vi "Create Image Saving Folder.vi"(0 "Camera Prime95B Controller in":refnum<class "Camera Prime95B Controller.lvclass">, 5 "Save Path":path, 7 "File suffix":string, 9 "StreamToDisk?":bool, 11 "error in (no error)":errorcluster) -> (4 "Camera Prime95B Controller out":refnum<class "Camera Prime95B Controller.lvclass">, 6 "Saving Path":path, 8 "Stream Saving Path":path, 15 "error out":errorcluster)   [LabVIEW 2020, in "Camera_Prime95B.lvlib" / "Camera Prime95B Controller.lvlib" / "Camera Prime95B Controller.lvclass"]
uses:
  Camera Prime95B Controller.lvclass
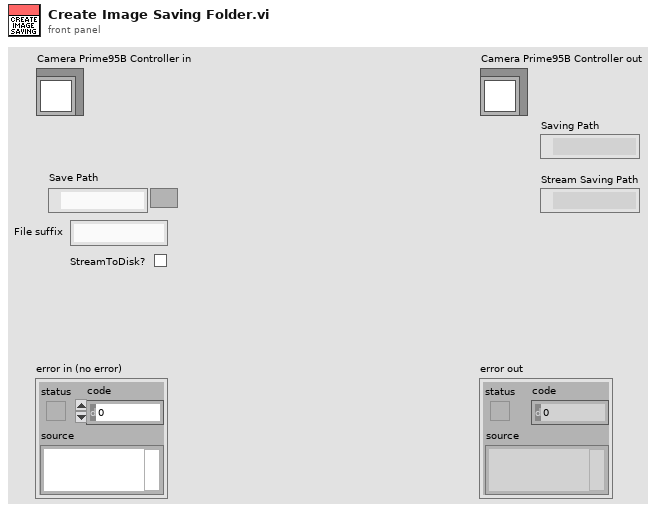
[diagram p1: front panel]
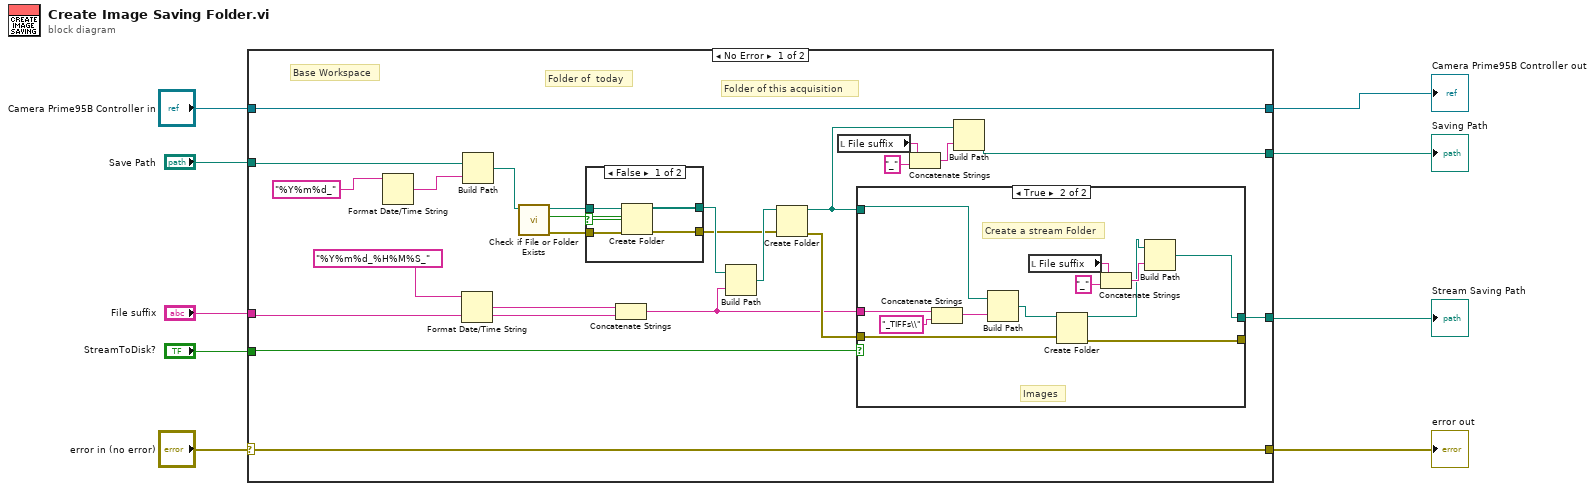
[diagram p0: block diagram]
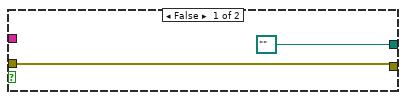
[diagram p2: hidden frame]
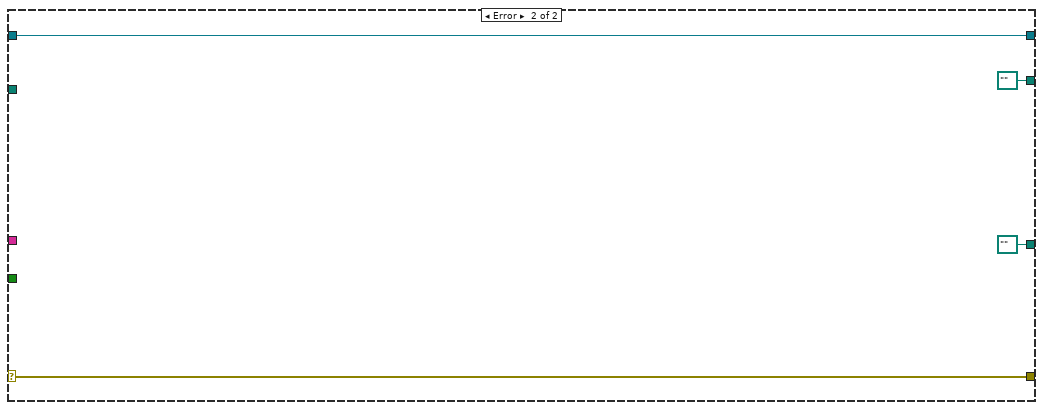
[diagram p4: hidden frame]
diagram:
  n1 = case shown="No Error" "error in (no error)" {
    selector: "error in (no error)" -> [w32 w57]
    tunnel: [w32 w57] -> w8
    tunnel: [w33 w56] -> w6
    tunnel: "Camera Prime95B Controller in" -> [w33 w56]
    tunnel: "Save Path" -> [w19 _]
    tunnel: "File suffix" -> [w18 _]
    tunnel: "StreamToDisk?" -> [w17 _]
    tunnel: [w15 path "" ("created path")] -> w1
    tunnel: [w13 path "" ("created path")] -> w2
    frame No Error {
      # "Base Workspace"
      # "Folder of this acquisition"
      # "Folder of  today"
      n2 = Format Date/Time String(time format string (%c)="%Y%m%d_") -> (date/time string=w22:string)  [unwired: 2 in]
      n3 = Format Date/Time String(time format string (%c)="%Y%m%d_%H%M%S_") -> (date/time string=w31:string)  [unwired: 2 in]
      n4 = Build Path(base path=w19, name or relative path=w22) -> (appended path=w23:path)
      n5 = call <vilib>:"Check if File or Folder Exists.vi"("path"=w23) -> ("error out"=w26:errorcluster, "file or folder exists?"=w24:bool, "dup path"=w25:path)  [unwired: 8 in]
      n6 = case shown="False" w24 {
        tunnel: w25 -> [w51 w53]
        tunnel: [w50 w52] -> w27
        tunnel: [w49 w53] -> w29
        tunnel: w26 -> [w48 w52]
        frame False {
          n7 = Create Folder(path (use dialog)=w51, error in=w48) -> (created path=w49:path, error out=w50:errorcluster)  [unwired: 1 in, 1 out]
        }
        frame True {
        }
      }
      n8 = Concatenate Strings(w31, w18) -> (w16:string)
      n9 = Build Path(base path=w29, name or relative path=w16) -> (appended path=w30:path)
      n10 = Create Folder(path (use dialog)=w30, error in=w27) -> (created path=w14:path, error out=w28:errorcluster)  [unwired: 1 in, 1 out]
      n11 = local read "File suffix"() -> (w12:string)
      n12 = case shown="True" w17 {
        tunnel: [path "" ("created path") w36] -> w15
        tunnel: w28 -> [w35 w47]
        tunnel: [w35 w46] -> _
        tunnel: w14 -> [_ w45]
        tunnel: w16 -> [_ w43]
        frame False {
        }
        frame True {
          # "Create a stream Folder"
          # "Images"
          n13 = Concatenate Strings(w43, "_TIFFs\\" ("string")) -> (w41:string)
          n14 = Build Path(base path=w45, name or relative path=w41) -> (appended path=w44:path)
          n15 = local read "File suffix"() -> (w38:string)
          n16 = Create Folder(path (use dialog)=w44, error in=w47) -> (created path=w37:path, error out=w46:errorcluster)  [unwired: 1 in, 1 out]
          n17 = Concatenate Strings(w38, "_" ("string")) -> (w39:string)
          n18 = Build Path(base path=w37, name or relative path=w39) -> (appended path=w36:path)
        }
      }
      n19 = Concatenate Strings(w12, "_" ("string")) -> (w11:string)
      n20 = Build Path(base path=w14, name or relative path=w11) -> (appended path=w13:path)
    }
    frame Error {
    }
  }
  "error out" <- w8
  "Camera Prime95B Controller out" <- w6
  "Saving Path" <- w2
  "Stream Saving Path" <- w1
